vi "Chirp Z Transform.vi"   [LabVIEW 2014, in "NI_AALPro.lvlib"]
doc: "Computes the Chirp-Z transform of the input sequence <B>X</B>. Wire data to the <B>X</B> input to determine the polymorphic instance to use or manually select the instance."
uses:
  NI_AALPro.lvlib
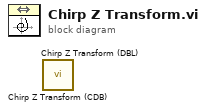
[diagram p0: block diagram]
diagram:
  n1 = call "Chirp Z Transform (CDB).vi"() -> ()  [unwired: 10 in, 2 out]
  n2 = call "Chirp Z Transform (DBL).vi"() -> ()  [unwired: 10 in, 2 out]
